vi "Palette.vi"(7 "Actor in":refnum<class "Actor.lvclass">, 10 "Spawn":refnum<class "Spawn.lvclass">) -> (0 "Error out":errorcluster, 5 "Actor out":refnum<class "Actor.lvclass">)   [LabVIEW 2025, in "jettl.lvlib" / "Transport.lvlib" / "Event.lvlib"]
uses:
  Event.lvlib
  Spawn/Spawn/Spawn.lvclass
  Actor/Actor.lvclass
  jettl.lvlib
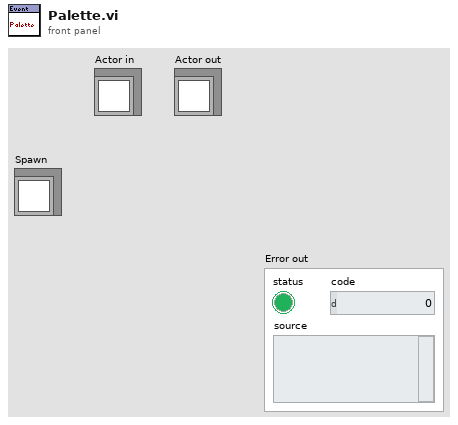
[diagram p1: front panel]
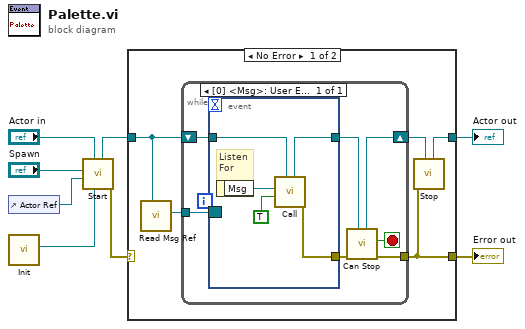
[diagram p0: block diagram]
diagram:
  n1 = control-ref of="Actor Ref"() -> (w5:refnum<vi>)
  n2 = call "Init.vi"() -> ("Transport"=w1:refnum<class "Transport.lvclass">)  [unwired: 11 in]
  n3 = call "Start.vi"("Transport"=w1, "Actor in"="Actor in", "Actor Ref"=w5, "Spawn"="Spawn") -> ("Error out"=w7:errorcluster, "Actor out"=w6:refnum<class "Actor.lvclass">)  [unwired: 6 in]
  n4 = case shown="No Error" w7 {
    selector: w7 -> [_ w26]
    tunnel: [w11 w27] -> w3
    tunnel: w6 -> [w10 w27]
    tunnel: [w13 w26] -> w8
    frame No Error {
      n5 = call "Read Msg Ref.vi"("Actor"=w10) -> ("Msg Ref"=w9:refnum<event-registration>)  [unwired: 10 in]
      n6 = while {
        shift-right: [w16] -> w12
        shift-left: w10 -> [w19]
        tunnel: w9 -> [w20]
        tunnel: [w17] -> w13
        stop <- w15 stop-if-true
        n7 = event shown="[0] <Msg>: User Event" {
          selector: w20 -> [_]
          dyn-events: _ -> [_]
          timeout: _ -> [_]
          tunnel: w19 -> [w25]
          tunnel: [w24] -> w14
          tunnel: [w22] -> w18
          event User Event {
            # "Listen\nFor"
            n8 = event-data() -> ("Msg"=w23:refnum<class "Msg.lvclass">)  [unwired: 1 in]
            n9 = call "Call.vi"("Actor in"=w25, "Listened To Msg"=TRUE, "Msg"=w23) -> ("Error out"=w22:errorcluster, "Actor out"=w24:refnum<class "Actor.lvclass">)  [unwired: 6 in, 1 out]
          }
        }
        n10 = call "Can Stop.vi"("Actor in"=w14, "Error in"=w18) -> ("Error out"=w17:errorcluster, "Stop"=w15:bool, "Actor out"=w16:refnum<class "Actor.lvclass">)  [unwired: 7 in]
      }
      n11 = call "Stop.vi"("Actor in"=w12, "Error in"=w13) -> ("Actor out"=w11:refnum<class "Actor.lvclass">)  [unwired: 9 in]
    }
    frame Error {
    }
  }
  "Error out" <- w8
  "Actor out" <- w3
